vi "HandleTx.vi"(8 "error in (no error)":errorcluster, 11 "Server in":refnum<class "Server.lvclass">) -> (0 "error out":errorcluster, 3 "Server out":refnum<class "Server.lvclass">)   [LabVIEW 2018, in "Server.lvclass"]
uses:
  Server.lvclass
  Server.lvclass/Server.ctl
  Comm/Stream/Stream.lvclass
panel:
  in  "MsgTX":string
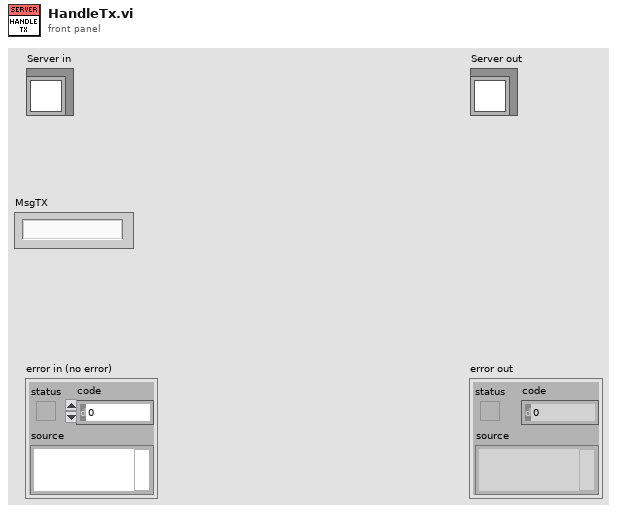
[diagram p1: front panel]
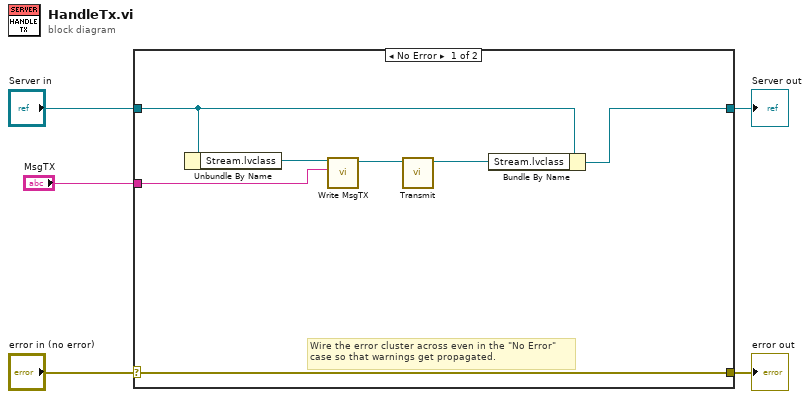
[diagram p0: block diagram]
diagram:
  n1 = case shown="No Error" "error in (no error)" {
    selector: "error in (no error)" -> [w12 w14]
    tunnel: [w12 w14] -> w4
    tunnel: [w6 w13] -> w2
    tunnel: "Server in" -> [w8 w13]
    tunnel: "MsgTX" -> [w11 _]
    frame No Error {
      # "Wire the error cluster across even in the \"No Error\"\ncase so that warnings get propagated."
      n2 = Unbundle By Name(w8) -> ("Stream.lvclass"=w10:refnum<class "Stream.lvclass">)
      n3 = call-dynamic "Write MsgTX.vi"("MsgTX"=w11, "Comm in"=w10) -> ("Comm out"=w9:refnum<class "Stream.lvclass">)  [unwired: 8 in, 1 out]
      n4 = call-dynamic "Transmit.vi"("Stream in"=w9) -> ("Stream out"=w7:refnum<class "Stream.lvclass">)  [unwired: 9 in, 1 out]
      n5 = Bundle By Name(cluster=w8, "Stream.lvclass"=w7) -> (w6:refnum<class "Server.lvclass">)
    }
    frame Error {
    }
  }
  "error out" <- w4
  "Server out" <- w2
